vi "保存mes.vi"(11 "参数值":T1(array[cluster])) -> (0 "error out":errorcluster, 3 "出站成功":bool)   [LabVIEW 2020]
uses:
  Global.vi
  <vilib>/Utility/file.llb/Write Delimited Spreadsheet (string).vi
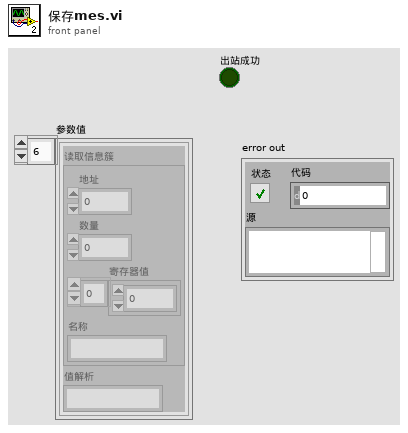
[diagram p1: front panel]
types:
  T1 = cluster{"读取信息簇":cluster{"地址":u16, "数量":u16, "寄存器值":u16[], "名称":string}, "值解析":string}[]
  T2 = cluster{"Server":string, "audit_mode":string, "tsid":string, "model":string, "product":string, "test_station":string, "station_id":string, "test_station_name":string, "Webservice":string}
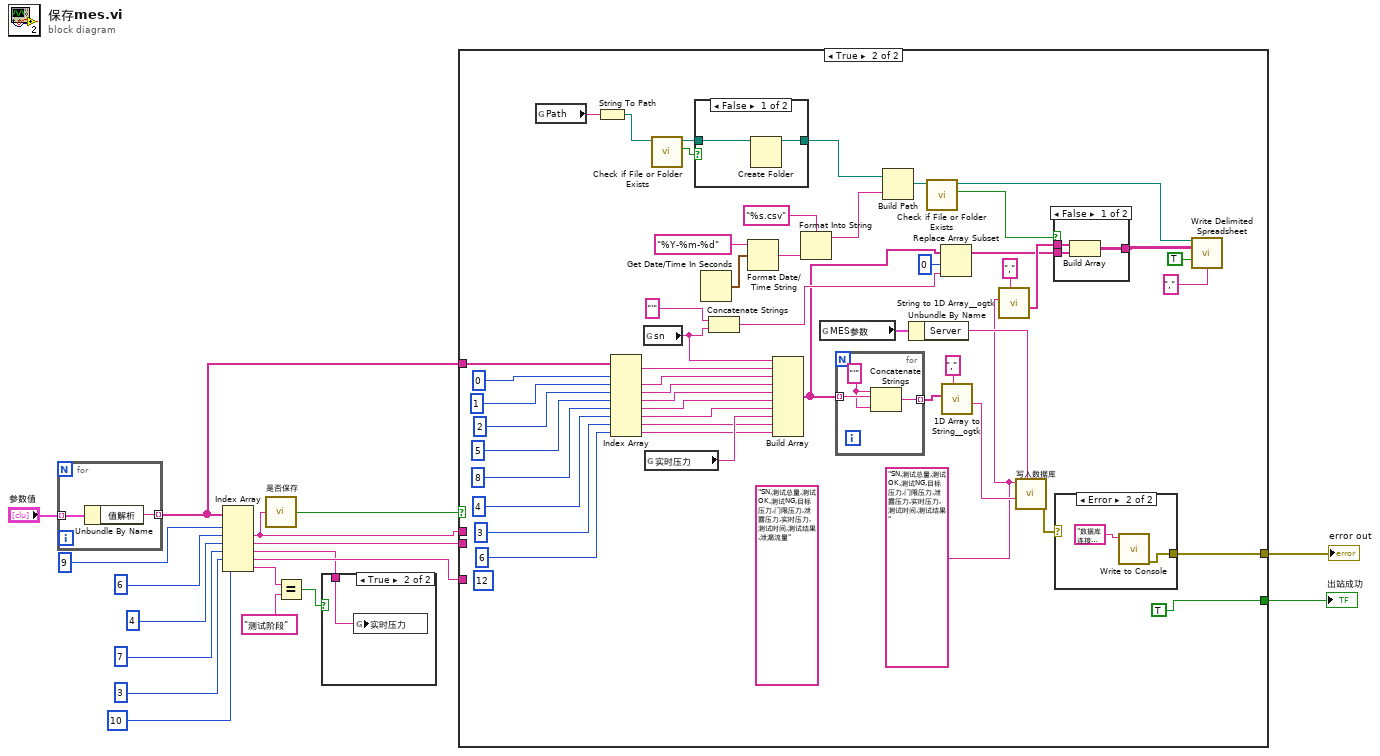
[diagram p0: block diagram]
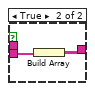
[diagram p4: hidden frame]
diagram:
  n1 = for {
    tunnel: "参数值" -> [w20] mode=indexing
    tunnel: [w19] -> w3 mode=indexing
    n2 = Unbundle By Name(w20) -> ("值解析"=w19:string)
  }
  n3 = Index Array(array=w3, index #1=9 ("索引"), index #2=6 ("索引"), index #3=4 ("索引"), index #4=7 ("索引"), index #5=3 ("索引"), index #6=10 ("索引")) -> (element #2=w13:string, element #3=w12:string, element #4=w4:string, element #5=w11:string, element #6=w7:string)  [unwired: 1 out]
  n4 = call "是否保存.vi"("测试结果"=w13) -> ("保存"=w10:bool)
  n5 = Equal?(x=w7, y="测试阶段") -> (x = y?=w5:bool)
  n6 = case shown="True" w5 {
    tunnel: w4 -> [_ w21]
    frame False {
    }
    frame True {
      n7 = global write "Global.vi" "实时压力"(w21) -> ()
    }
  }
  n8 = case shown="True" w10 {
    tunnel: w13 -> [_ _]
    tunnel: w12 -> [_ _]
    tunnel: w11 -> [_ _]
    tunnel: w3 -> [_ w72]
    tunnel: [_ w50] -> w2
    tunnel: [_ TRUE] -> w1
    frame False {
    }
    frame True {
      (unwired) "SN,测试总量,测试OK,测试NG,目标压力,门限压力,泄露压力,实时压力,测试时间,测试结果,泄漏流量" ("测量项目")
      w33 = "SN,测试总量,测试OK,测试NG,目标压力,门限压力,泄露压力,实时压力,测试时间,测试结果" ("测量项目")
      (unwired) 12 ("索引")
      n9 = global read "Global.vi" "Path"() -> (w39:string)
      n10 = String To Path(string=w39) -> (path=w38:path)
      n11 = Index Array(array=w72, index #1=0 ("索引"), index #2=1 ("索引"), index #3=2 ("索引"), index #4=5 ("索引"), index #5=8 ("索引"), index #6=4 ("索引"), index #7=3 ("索引"), index #8=6 ("索引")) -> (element #1=w63:string, element #2=w62:string, element #3=w61:string, element #4=w60:string, element #5=w59:string, element #6=w58:string, element #7=w56:string, element #8=w55:string)
      n12 = global read "Global.vi" "sn"() -> (w25:string)
      n13 = global read "Global.vi" "实时压力"() -> (w57:string)
      n14 = call <vilib>:"Check if File or Folder Exists.vi"("path"=w38) -> ("file or folder exists?"=w43:bool, "dup path"=w42:path)  [unwired: 8 in, 1 out]
      n15 = case shown="False" w43 {
        tunnel: w42 -> [w79 w80]
        tunnel: [w78 w80] -> w41
        frame False {
          n16 = Create Folder(path (use dialog)=w79) -> (created path=w78:path)  [unwired: 2 in, 2 out]
        }
        frame True {
        }
      }
      n17 = Get Date/Time In Seconds() -> (seconds since 1Jan1904=w46:timestamp)
      n18 = Concatenate Strings("'", w25) -> (w24:string)
      n19 = Format Date/Time String(time format string (%c)="%Y-%m-%d" ("时间格式字符串(%c)"), seconds (now)=w46) -> (date/time string=w45:string)  [unwired: 1 in]
      n20 = Build Array(w25, w63, w62, w61, w60, w59, w58, w57, w56, w55) -> (w22:string[])
      n21 = Format Into String(format string="%s.csv" ("格式字符串"), w45) -> (resulting string=w44:string)  [unwired: 2 in, 1 out]
      n22 = global read "Global.vi" "MES参数"() -> (w48:T2)
      n23 = for {
        tunnel: w22 -> [w86] mode=indexing
        tunnel: [w84] -> w53 mode=indexing
        w85 = "'"
        n24 = Concatenate Strings(w85, w86, w85) -> (w84:string)
      }
      n25 = Build Path(base path=w41, name or relative path=w44) -> (appended path=w40:path)
      n26 = Unbundle By Name(w48) -> ("Server"=w47:string)
      n27 = call <vilib>:"Check if File or Folder Exists.vi"("path"=w40) -> ("file or folder exists?"=w37:bool, "dup path"=w28:path)  [unwired: 8 in, 1 out]
      n28 = Replace Array Subset(array=w22, new element=w24, index=0) -> (w23:string[])
      n29 = call <userlib>:"1D Array to String__ogtk.vi"("delimiter (Tab)"=",", "Array of Strings"=w53) -> ("delimited string"=w52:string)  [unwired: 9 in]
      n30 = call <userlib>:"String to 1D Array__ogtk.vi"("delimiter (Tab)"=",", "string"=w33) -> ("Array of Strings"=w32:string[])  [unwired: 9 in]
      n31 = call "写入数据库.vi"("SERVER(IP)"=w47, "values"=w52, "测试项目"=w33) -> ("error out"=w51:errorcluster)  [unwired: 8 in]
      n32 = case shown="False" w37 {
        tunnel: w32 -> [w75 _]
        tunnel: w23 -> [w74 w77]
        tunnel: [w73 w76] -> w29
        frame False {
          n33 = Build Array(w75, w74) -> (w73:string[][])
        }
        frame True {
          n34 = Build Array(w77) -> (w76:string[][])
        }
      }
      n35 = case shown="Error" w51 {
        selector: w51 -> [w81 _]
        tunnel: [w81 w82] -> w50
        frame No Error {
        }
        frame Error {
          n36 = call "Write to Console.vi"("Input"="数据库连接错误。" ("消息")) -> ("error out"=w82:errorcluster)  [unwired: 10 in]
        }
      }
      n37 = call-poly <vilib>:"Write Delimited Spreadsheet.vi"("file path (dialog if empty)"=w28, "2D data"=w29, "append to file? (new file:F)"=TRUE ("append to file? (F)"), "delimiter (\\t)"="," ("delimiter (\\t)")) -> ()  [unwired: 10 in, 2 out]
    }
  }
  "出站成功" <- w1
  "error out" <- w2
